vi "status.vi"(3 "error in (no error)":errorcluster, 5 "HGF_SVMonitor":refnum<class "HGF_SVMonitor.lvclass">) -> (0 "error out":errorcluster, 1 "Array":T1(array[cluster]), 2 "dup HGF_SVMonitor":refnum<class "HGF_SVMonitor.lvclass">)   [LabVIEW 2012, in "HGF_SV.lvlib" / "HGF_SVMonitor.lvclass"]
doc: "Request status from monitor"
uses:
  HGF_SVMonitor.lvclass
  HGF_BaseClasses/HGF_NetworkVisitor/HGF_NetworkVisitor.lvclass
  HGF_BaseClasses/HGF_TriggeredEvent/HGF_TriggeredEvent.lvclass
  <resource>/objmgr/ni.var.rc
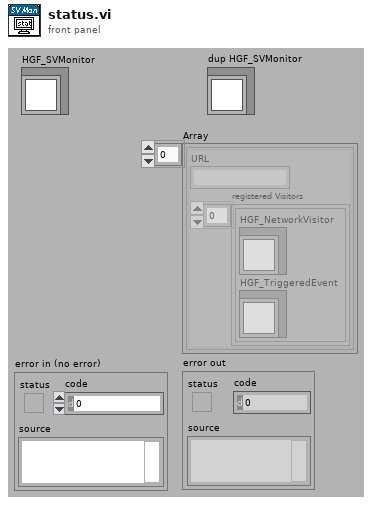
[diagram p1: front panel]
types:
  T1 = cluster{"URL":string, "registered Visitors":cluster{"HGF_NetworkVisitor":refnum<class "HGF_NetworkVisitor.lvclass">, "HGF_TriggeredEvent":refnum<class "HGF_TriggeredEvent.lvclass">}[]}[]
  T2 = cluster{"registered Visitors":cluster{"HGF_NetworkVisitor":refnum<class "HGF_NetworkVisitor.lvclass">, "HGF_TriggeredEvent":refnum<class "HGF_TriggeredEvent.lvclass">}[], "last known data":variant, "Time Stamp":timestamp, "shared variable refnum in":refnum<k21>}[]
  T3 = cluster{"HGF_NetworkVisitor":refnum<class "HGF_NetworkVisitor.lvclass">, "HGF_TriggeredEvent":refnum<class "HGF_TriggeredEvent.lvclass">}[]
  T4 = cluster{"URL":string, "registered Visitors":cluster{"HGF_NetworkVisitor":refnum<class "HGF_NetworkVisitor.lvclass">, "HGF_TriggeredEvent":refnum<class "HGF_TriggeredEvent.lvclass">}[]}
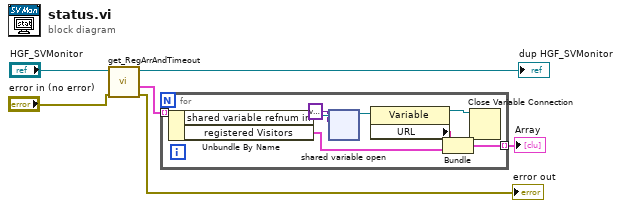
[diagram p0: block diagram]
diagram:
  n1 = call "get_RegArrAndTimeout.vi"("error in (no error)"="error in (no error)", "HGF_SVMonitor"="HGF_SVMonitor") -> ("error out"=→"error out":errorcluster, "Registration Array"=w2:T2, "HGF_SVMonitor"=→"dup HGF_SVMonitor":refnum<class "HGF_SVMonitor.lvclass">)  [unwired: 2 in, 1 out]
  n2 = for {
    tunnel: w2 -> [w14] mode=indexing
    tunnel: [w12] -> w1 mode=indexing
    n3 = Unbundle By Name(w14) -> ("shared variable refnum in"=w11:refnum<k21>, "registered Visitors"=w13:T3)
    n4 = shared-variable-open(w11, variant ("variant")) -> (w10:refnum<k21>)  [unwired: 2 in, 1 out]
    n5 = property class="Variable"(reference=w10) -> (reference out=w9:refnum<k21>, "URL"=w8:string)  [unwired: 1 in, 1 out]
    n6 = Bundle("URL"=w8, "registered Visitors"=w13) -> (w12:T4)  [unwired: 1 in]
    n7 = Close Variable Connection(11:w9) -> ()  [unwired: 1 in, 1 out]
  }
  "Array" <- w1
